vi "Read PythonVersion.vi"(8 "error in (no error)":errorcluster, 11 "PythonWrapper in":refnum<class "PythonWrapper.lvclass">) -> (0 "error out":errorcluster, 2 "PythonVersion":string="3.9", 3 "PythonWrapper out":refnum<class "PythonWrapper.lvclass">)   [LabVIEW 2022 SP3, in "PythonWrapper.lvlib" / "PythonWrapper.lvclass"]
uses:
  PythonWrapper.lvclass
  PythonWrapper.lvclass/PythonWrapper.ctl
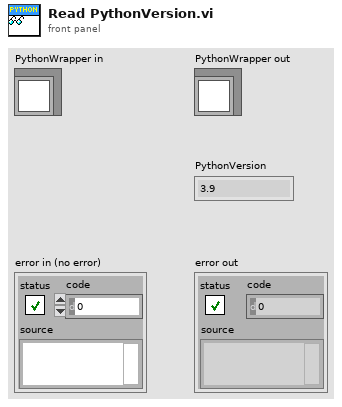
[diagram p1: front panel]
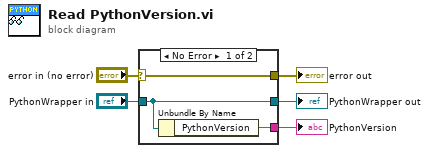
[diagram p0: block diagram]
diagram:
  n1 = case shown="No Error" "error in (no error)" {
    selector: "error in (no error)" -> [w8 w9]
    tunnel: [w8 w9] -> w4
    tunnel: [w7 w10] -> w2
    tunnel: "PythonWrapper in" -> [w7 w10]
    tunnel: [w6 _] -> w1
    frame No Error {
      n2 = Unbundle By Name(w7) -> ("PythonVersion"=w6:string)
    }
    frame Error {
    }
  }
  "error out" <- w4
  "PythonWrapper out" <- w2
  "PythonVersion" <- w1
